vi "Load_Info.vi"(8 "error in (no error)":errorcluster, 11 "AB_Deploy_EXE in":refnum<class "AB_Deploy_EXE.lvclass">) -> (0 "error out":errorcluster, 3 "AB_Deploy_EXE out":refnum<class "AB_Deploy_EXE.lvclass">)   [LabVIEW 2020, in "AB_Deploy_EXE.lvclass"]
uses:
  <vilib>/AppBuilder/AB_Classes/DeployableEXE/AB_Deploy_EXE.lvclass
  e:/builds/penguin/labview/branches/2020/dev/dist/vi.lib/AppBuilder/AB_Classes/Build/AB_Build.lvclass
  <vilib>/AppBuilder/RW_Project/AB_RW_Project_PropBag_Action.ctl
  <vilib>/AppBuilder/AB_Classes/DeployableEXE/AB_Deploy_EXE.lvclass/AB_Deploy_EXE.ctl
  <vilib>/AppBuilder/AB_Classes/EXE/AB_EXE.lvclass
  <vilib>/AppBuilder/AB_Classes/Build/AB_Build.lvclass
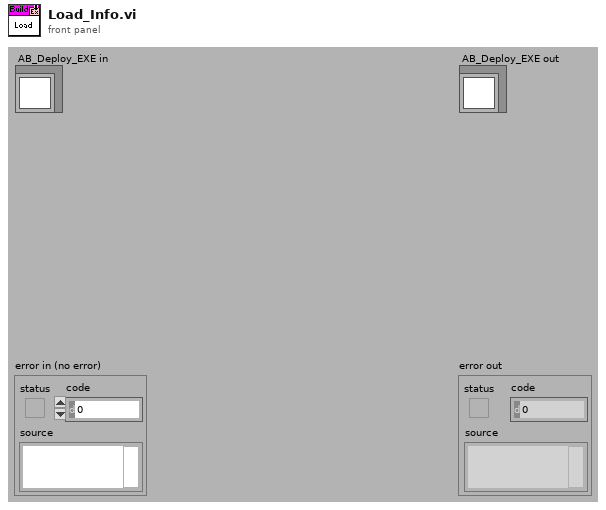
[diagram p1: front panel]
types:
  T1 = typedef "AB_RW_Project_PropBag_Action.ctl" = enum16{"read", "write", "clear", "readPrevious", "writePrevious", "clearPrevious"}
  T2 = typedef "AB_Build.ctl" = cluster{"buildSpecName":string, "buildSpecDescription":string, "destinations":refnum<class "AB_Destination.lvclass">[], "exclusionOption":T3, "defaultLanguage":string, "supportedLanguages":string[], "excludedDirectories":path[], "buildContext":refnum<vi>, "buildObject":T4, "preview":bool, "programatic":bool, "progressBarEvents":T5, "userLog_Path":path, "preActionID":string, "preAction_Path":path, "postActionID":string, "postAction_Path":path, "eng_checkForBrokenVIs?":bool, "eng_verboseLinkerErrors?":bool, "localDest_Path":path, "targetDest_Path":path, "removeVIObject":u16, "cache":refnum<class "PreviewCache.lvclass">, "use cache":bool, "previewCache_ID":string, "buildCache_ID":string, "eng_TempLocalDest_Path":path, "eng_collectDependencies?":bool, "versionInfo":cluster{"buildVersion":cluster{"major":u16, "minor":u16, "patch":u16, "build":u16}, "autoIncrement":bool}, "eng_enableVIChecksums":bool}
  T3 = typedef "AB_Exclusion_Option.ctl" = cluster{"typedefs":bool, "polymorphicVIs":bool, "unusedLibraryItems":bool, "modifyLibraryFile":bool, "edit-timeDependencies":bool, "inlineVIs":bool, "dependent PPLs":bool, "dependent DLLs":bool}
  T4 = typedef "ItemRef.ctl" = u64
  T5 = typedef "provcom_ProgressBar_Events.ctl" = cluster{"newJob":refnum<user-event>, "newItem":refnum<user-event>, "errorMsg":T6, "cancel":refnum<user-event>}
  T6 = typedef "mxLvBuildError.ctl" = refnum<user-event>
  T7 = typedef "AB_RW_Project_Deploy_EXE_Data.ctl" = cluster{"localDestPath":path}
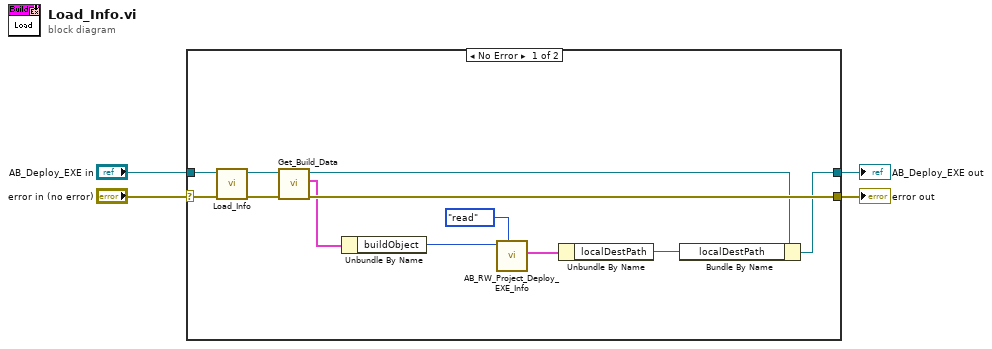
[diagram p0: block diagram]
diagram:
  n1 = case shown="No Error" "error in (no error)" {
    selector: "error in (no error)" -> [w15 w17]
    tunnel: [w12 w17] -> w4
    tunnel: [w10 w18] -> w3
    tunnel: "AB_Deploy_EXE in" -> [w16 w18]
    frame No Error {
      n2 = call-parent "Load_Info.vi"("error in (no error)"=w15, "AB_EXE in"=w16) -> ("error out"=w13:errorcluster, "AB_EXE out"=w14:refnum<class "AB_Deploy_EXE.lvclass">)  [unwired: 8 in]
      n3 = call <vilib>:"Get_Build_Data.vi"("error in (no error)"=w13, "Class in"=w14) -> ("error out"=w12:errorcluster, "data"=w11:T2, "Class out"=w9:refnum<class "AB_Deploy_EXE.lvclass">)  [unwired: 7 in]
      n4 = Unbundle By Name(w11) -> ("buildObject"=w5:T4)
      n5 = call <vilib>:"AB_RW_Project_Deploy_EXE_Info.vi"("action"=AB_RW_Project_PropBag_Action."read", "Object In"=w5) -> ("info out"=w8:T7)  [unwired: 7 in, 2 out]
      n6 = Unbundle By Name(w8) -> ("localDestPath"=w6:path)
      n7 = Bundle By Name(cluster=w9, "localDestPath"=w6) -> (w10:refnum<class "AB_Deploy_EXE.lvclass">)
    }
    frame Error {
    }
  }
  "error out" <- w4
  "AB_Deploy_EXE out" <- w3
